vi "Update_Table_Value.vi"(1 "Mode":T2(ring), 2 "Update array in":T1[](array[typedef]) {"New Value" format="%.2f"}) -> (0 "Update array out":T1[](array[typedef]) {"New Value" format="%.2f"})   [LabVIEW 2010]
uses:
  ADAM Client/Sub VIs/ADAM Controls/Update_scan_value.ctl
  ADAM_Global.vi
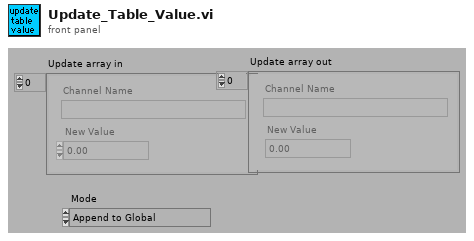
[diagram p1: front panel]
types:
  T1 = typedef "Update_scan_value.ctl" = cluster{"Channel Name":string, "New Value":dbl}
  T2 = enum16{"Append to Global", "Read Global then Clear"}
  T3 = cluster{"Channel Name":string, "New Value":dbl}[]
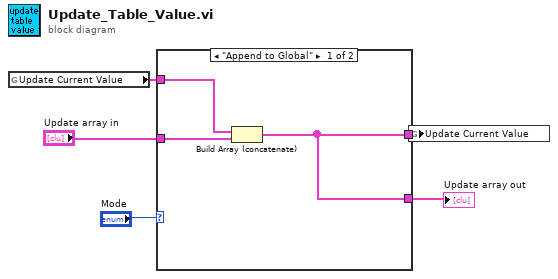
[diagram p0: block diagram]
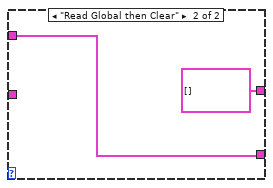
[diagram p2: hidden frame]
diagram:
  n1 = global read "ADAM_Global.vi" "Update Current Value"() -> (w5:T1[])
  n2 = case shown="\"Append to Global\"" "Mode" {
    tunnel: w5 -> [w8 w10]
    tunnel: "Update array in" -> [w7 _]
    tunnel: [w6 T3 []] -> w2
    tunnel: [w6 w10] -> w1
    frame "Append to Global" {
      n3 = Build Array (concatenate)(w8, w7) -> (w6:T1[])
    }
    frame "Read Global then Clear" {
    }
  }
  "Update array out" <- w1
  n4 = global write "ADAM_Global.vi" "Update Current Value"(w2) -> ()
